vi "waveform1.vi"() -> ()   [LabVIEW 2021]
panel:
  out "Max":dbl
  out "duration":dbl
  out "Min":dbl
  out "Waveform Graph":waveform(dbl)(graph)
  in  "# of Points":i64
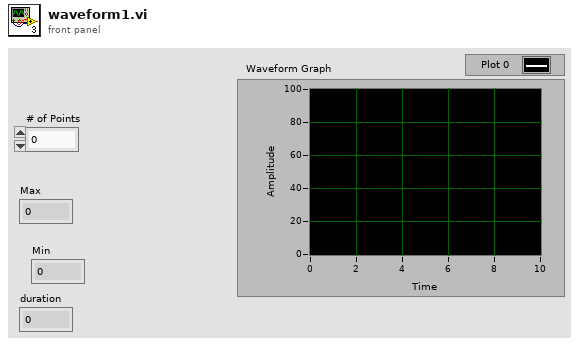
[diagram p1: front panel]
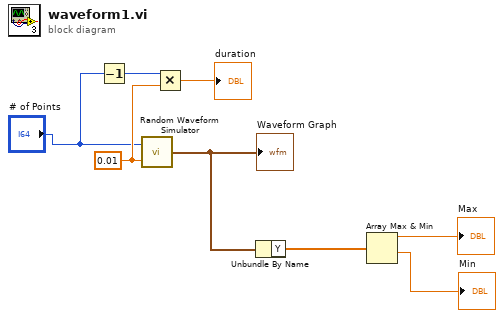
[diagram p0: block diagram]
diagram:
  w4 = 0.01
  n1 = Decrement(x="# of Points") -> (x-1=w1:i64)
  n2 = call "Random Waveform Simulator.vi"("dt"=w4, "# Points"="# of Points") -> ("waveform out"=w8:waveform(dbl))  [unwired: 1 in]
  "Waveform Graph" <- w8
  n3 = Multiply(x=w1, y=w4) -> (x*y=→"duration":dbl)
  n4 = Unbundle By Name(w8) -> ("Y"=w7:dbl[])
  n5 = Array Max & Min(array=w7) -> (max value=→"Max":dbl, min value=→"Min":dbl)  [unwired: 2 out]
